vi "checkchanged.vi"(11 "mode":variant) -> (3 "Boolean":bool)   [LabVIEW 2017, in "UI_TimeSelector.xctl"]
uses:
  UI_TimeSelector.xctl
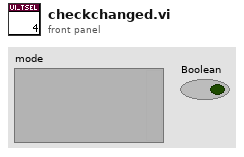
[diagram p1: front panel]
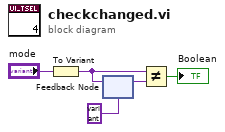
[diagram p0: block diagram]
diagram:
  n1 = To Variant(anything="mode") -> (Variant=w3:variant)
  n2 = feedback #1(variant ("Variant")) -> (w1:variant)
  n3 = feedback-in #1(w3) -> ()
  n4 = Not Equal?(x=w3, y=w1) -> (x != y?=→"Boolean":bool)
